vi "OCR_Characterize Columns.vi"(7 "Color Set":T1={"BG"=255, "FG"=16711680}, 8 "Error":errorcluster, 11 "2D Image":u32[][](array[colorbox])) -> (0 "Error Out":errorcluster, 3 "Column Type Aray Out":T2[](array[typedef]))   [LabVIEW 2009]
doc: "Determines the column type of each column in the 2D image"
uses:
  Controls/Enum/ENUM_Line Letter Type.ctl
  Controls/Cluster/Cluster_Text Color Set.ctl
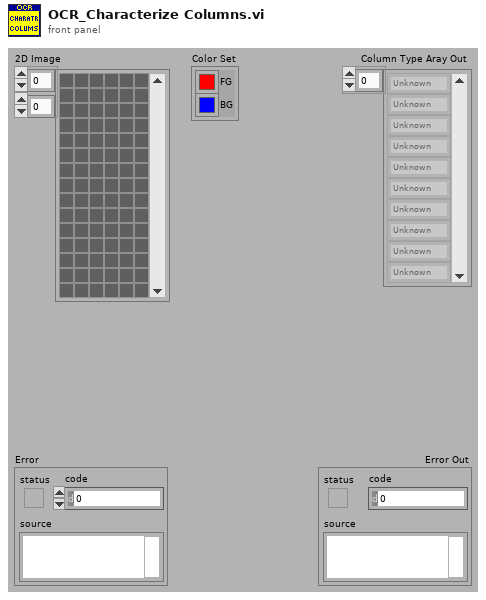
[diagram p1: front panel]
types:
  T1 = typedef "Cluster_Text Color Set.ctl" = cluster{"BG":u32, "FG":u32}
  T2 = typedef "ENUM_Line Letter Type.ctl" = enum16{"Unknown", "Letter", "Seperator", "Seperator or Letter"}
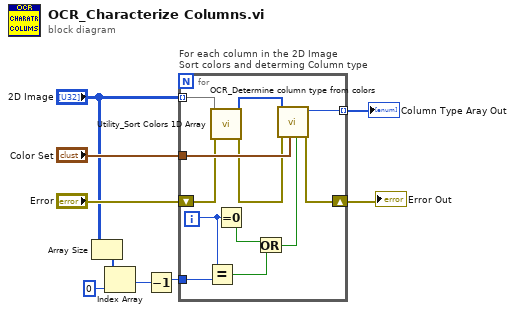
[diagram p0: block diagram]
diagram:
  n1 = Array Size(array="2D Image") -> (size(s)=w4:i32[])
  n2 = Index Array(array=w4, index=0) -> (element=w3:i32)
  n3 = Decrement(x=w3) -> (x-1=w2:i32)
  n4 = for "For each column in the 2D Image\nSort colors and determing Column type" {
    tunnel: "2D Image" -> [w18] mode=indexing
    tunnel: [w20] -> w9 mode=indexing
    shift-right: [w21] -> w8
    shift-left: "Error" -> [w16]
    tunnel: "Color Set" -> [w19]
    tunnel: w2 -> [w14]
    i -> [w13]
    n5 = Equal?(x=w13, y=w14) -> (x = y?=w11:bool)
    n6 = call "Utility_Sort Colors 1D Array.vi"("Error"=w16, "Colors"=w18) -> ("Error Out"=w15:errorcluster, "Sorted By Quantity Out"=w17:u32[])  [unwired: 7 in, 1 out]
    n7 = Equal To 0?(x=w13) -> (x = 0?=w12:bool)
    n8 = Or(x=w12, y=w11) -> (x .or. y?=w10:bool)
    n9 = call "OCR_Determine column type from colors.vi"("Seperator Or Letter If Solid"=w10, "Color Set"=w19, "Error"=w15, "Color List"=w17) -> ("Error Out"=w21:errorcluster, "Type Out"=w20:T2)  [unwired: 6 in]
  }
  "Column Type Aray Out" <- w9
  "Error Out" <- w8
